vi "Pass Ref and Receive Data.vi"(7 "Enum":T4=enum."Pass Data", 8 "error in (no error)":errorcluster, 10 "Data":T2={"Raw Data"=[], "Volt Channel"={"Index"=[], "Chl Name"=[], "Scale"=[], "Offset"=[], "Sample Rate"=100, "Device Name"="", "Channel"=""}}, 11 "Chart in":refnum<class "Chart.lvclass">) -> (0 "error out":errorcluster, 3 "Chart out":refnum<class "Chart.lvclass">)   [LabVIEW 2021, in "Chart.lvclass"]
doc: "This vi has two functions:\nInitialize - Hold This VI reference in class. Clear chart history and enable Choose Formula \nPass Data - Display data on chart with raw data or conditioned data.s"
uses:
  Chart.lvclass
  Graph Abstract Class/Pass Ref and Receive Data -- Enum.ctl
  Graph Abstract Class/Graph Data -- cluster.ctl
  Control/Volt Chl.ctl
  Graph Abstract Class/Conditioned Formula  -- Enum.ctl
  Chart.lvclass/Chart.ctl
panel:
  in  "Choose Formula":T1 caption="Choose Formula Applied to the Raw Data"
  out "Waveform Chart":waveform(dbl)[](graph)
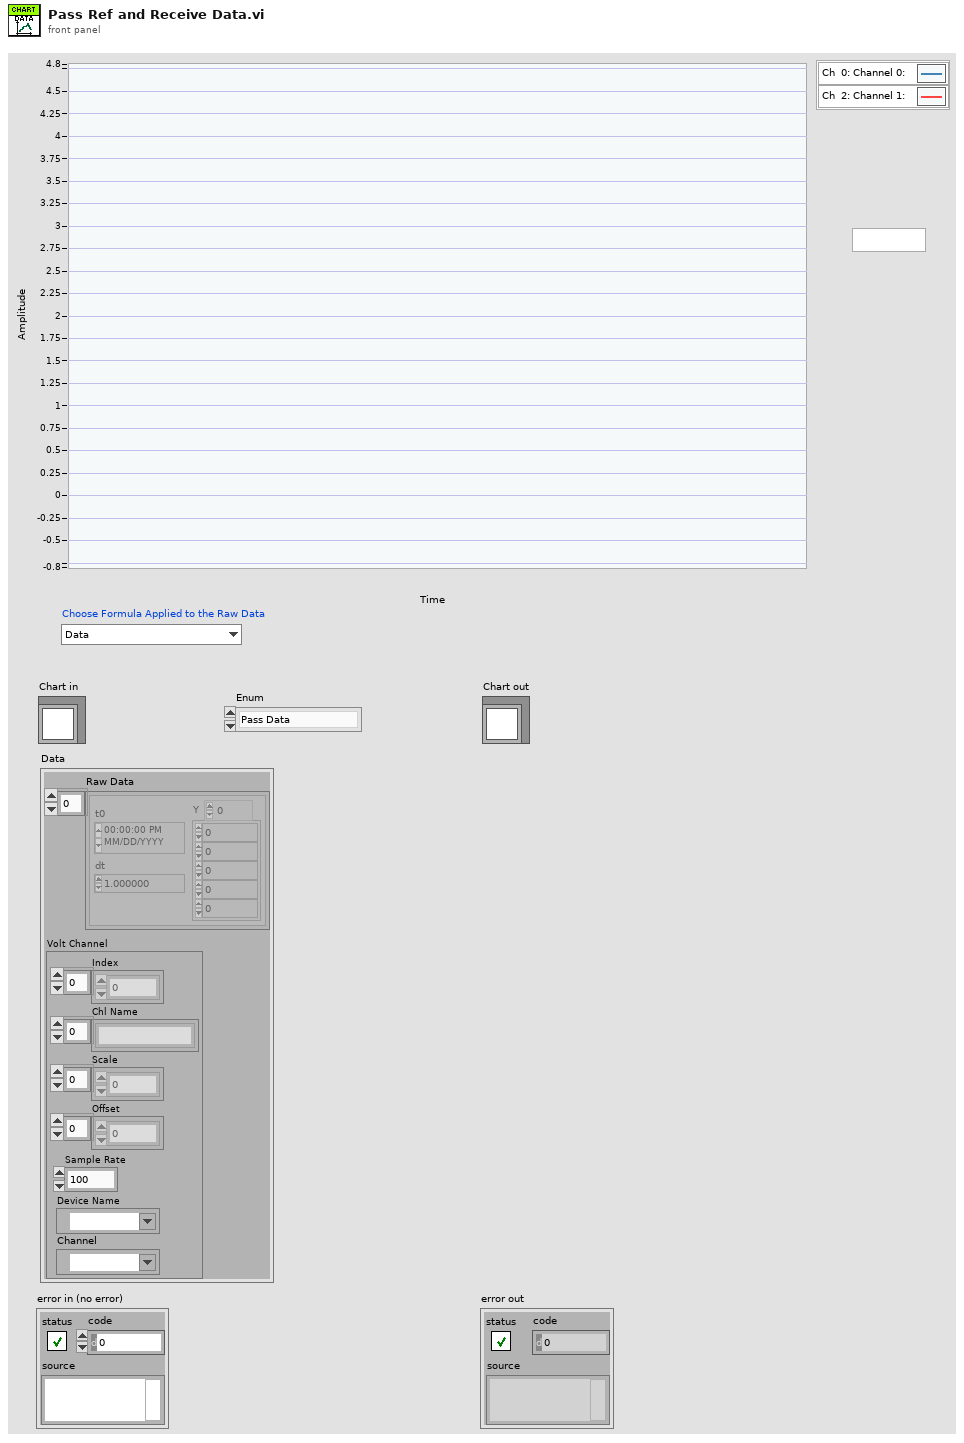
[diagram p1: front panel]
types:
  T1 = typedef "Conditioned Formula  -- Enum.ctl" = enum16{"Data", "Data*Scale+Offset"}
  T2 = typedef "Graph Data -- cluster.ctl" = cluster{"Raw Data":waveform(dbl)[], "Volt Channel":T3}
  T3 = typedef "Volt Chl.ctl" = cluster{"Index":i32[], "Chl Name":string[], "Scale":dbl[], "Offset":dbl[], "Sample Rate":i32, "Device Name":tag, "Channel":tag}
  T4 = typedef "Pass Ref and Receive Data -- Enum.ctl" = enum16{"Initialize", "Pass Data"}
  T5 = enum8{"Enabled", "Disabled", "Disabled and Grayed Out"}
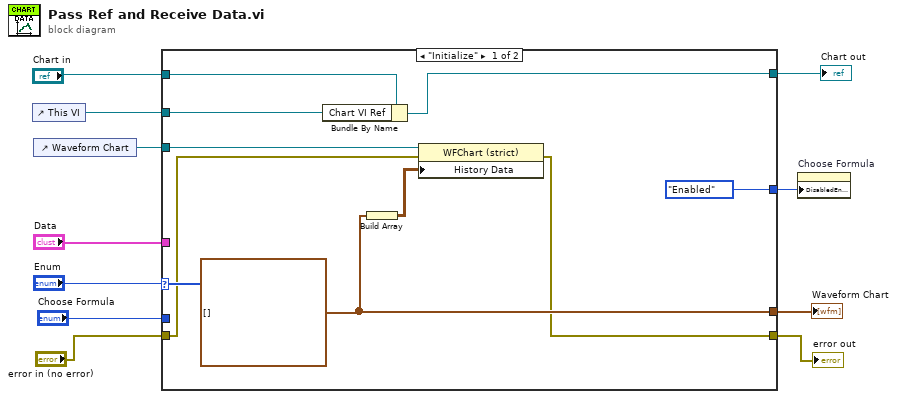
[diagram p0: block diagram]
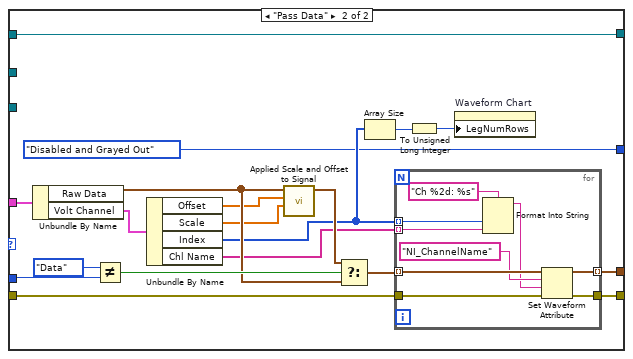
[diagram p2: hidden frame]
diagram:
  n1 = control-ref of="This VI"() -> (w9:refnum<vi>)
  n2 = control-ref of="Waveform Chart"() -> (w7:refnum<vi>)
  n3 = case shown="\"Initialize\"" "Enum" {
    tunnel: "Chart in" -> [w20 w38]
    tunnel: [w18 w38] -> w10
    tunnel: w9 -> [w19 _]
    tunnel: w7 -> [w16 _]
    tunnel: "Data" -> [_ w39]
    tunnel: [w15 w31] -> w5
    tunnel: "Choose Formula" -> [_ w35]
    tunnel: [T5."Enabled" ("Disabled") T5."Disabled and Grayed Out" ("Disabled")] -> w1
    tunnel: "error in (no error)" -> [w13 w30]
    tunnel: [w12 w29] -> w3
    frame "Initialize" {
      w15 = waveform(dbl)[] [] ("Raw Data")
      n4 = Bundle By Name(cluster=w20, "Chart VI Ref"=w19) -> (w18:refnum<class "Chart.lvclass">)
      n5 = Build Array(w15) -> (w14:waveform(dbl)[][])
      n6 = property class="WFChart (strict)"(reference=w16, error in=w13, "History Data"=w14) -> (error out=w12:errorcluster)  [unwired: 1 out]
    }
    frame "Pass Data" {
      n7 = Unbundle By Name(w39) -> ("Raw Data"=w34:waveform(dbl)[], "Volt Channel"=w28:T3)
      n8 = Not Equal?(x=Conditioned_Formula__--_Enum."Data", y=w35) -> (x != y?=w36:bool)
      n9 = Unbundle By Name(w28) -> ("Offset"=w27:dbl[], "Scale"=w26:dbl[], "Index"=w23:i32[], "Chl Name"=w25:string[])
      n10 = call "Applied Scale and Offset to Signal.vi"("Scale"=w26, "Offset"=w27, "Raw Data"=w34) -> ("Conditioned Signal"=w33:waveform(dbl)[])  [unwired: 8 in]
      n11 = Select(t=w33, s=w36, f=w34) -> (s? t:f=w32:waveform(dbl)[])
      n12 = Array Size(array=w23) -> (size(s)=w24:i32)
      n13 = for {
        tunnel: w32 -> [w48] mode=indexing
        tunnel: [w47] -> w31 mode=indexing
        tunnel: w30 -> [w45]
        tunnel: [w44] -> w29
        tunnel: w23 -> [w41] mode=indexing
        tunnel: w25 -> [w40] mode=indexing
        n14 = Format Into String(format string="Ch %2d: %s", w41, w40) -> (resulting string=w42:string)  [unwired: 2 in, 1 out]
        n15 = Set Waveform Attribute(4:w45, 5:w42, 6:"NI_ChannelName" ("name"), 7:w48) -> (0:w44:errorcluster, 3:w47:waveform(dbl))  [unwired: 1 out]
      }
      n16 = To Unsigned Long Integer(number=w24) -> (unsigned 32bit integer=w22:u32)
      n17 = property on="Waveform Chart" class="WFChart (strict)"("LegNumRows"=w22) -> ()  [unwired: 2 in, 2 out]
    }
  }
  "error out" <- w3
  "Chart out" <- w10
  "Waveform Chart" <- w5
  n18 = property on="Choose Formula" class="Enum (strict)"("DisabledEnum"=w1) -> ()  [unwired: 2 in, 2 out]
